vi "InitializeGenericCommandDialog.vi"(8 "Error In":errorcluster, 10 "Initial List Values":string[](array[string]), 11 "Dialog Enter Generic_UICtrlRefnums":T1) -> (0 "Error Out":errorcluster)   [LabVIEW 2012]
doc: "SciScan 1.2 160622"
uses:
  Dialog Enter Generic_UICtrlRefnums.ctl
  Custom Controls and Typedefs/BOOL Enum.ctl
  Custom Controls and Typedefs/Delete Button.ctl
  CommonResource VIs/UI Control and Indicator properties_Commands.ctl
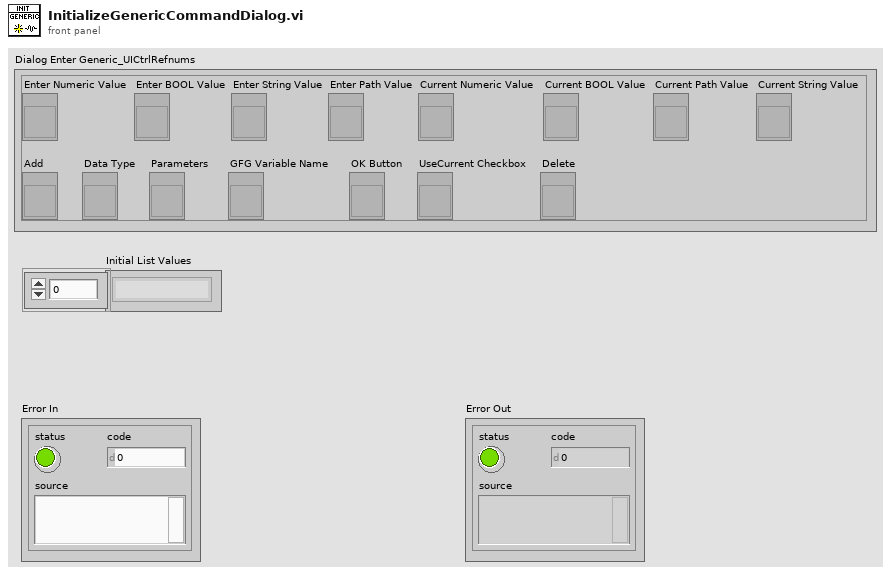
[diagram p1: front panel]
types:
  T1 = typedef "Dialog Enter Generic_UICtrlRefnums.ctl" = cluster{"Enter Numeric Value":refnum<vi>, "Enter BOOL Value":refnum<vi>, "Enter String Value":refnum<vi>, "Enter Path Value":refnum<vi>, "Add":refnum<vi>, "Data Type":refnum<vi>, "Parameters":refnum<vi>, "GFG Variable Name":refnum<vi>, "OK Button":refnum<vi>, "Current Numeric Value":refnum<vi>, "Current BOOL Value":refnum<vi>, "Current String Value":refnum<vi>, "Current Path Value":refnum<vi>, "UseCurrent Checkbox":refnum<vi>, "Delete":refnum<vi>}
  T2 = typedef "UI Control and Indicator properties_Commands.ctl" = enum16{"Enable", "Disable", "Disable and Grey", "Make Visible", "Make Invisible"}
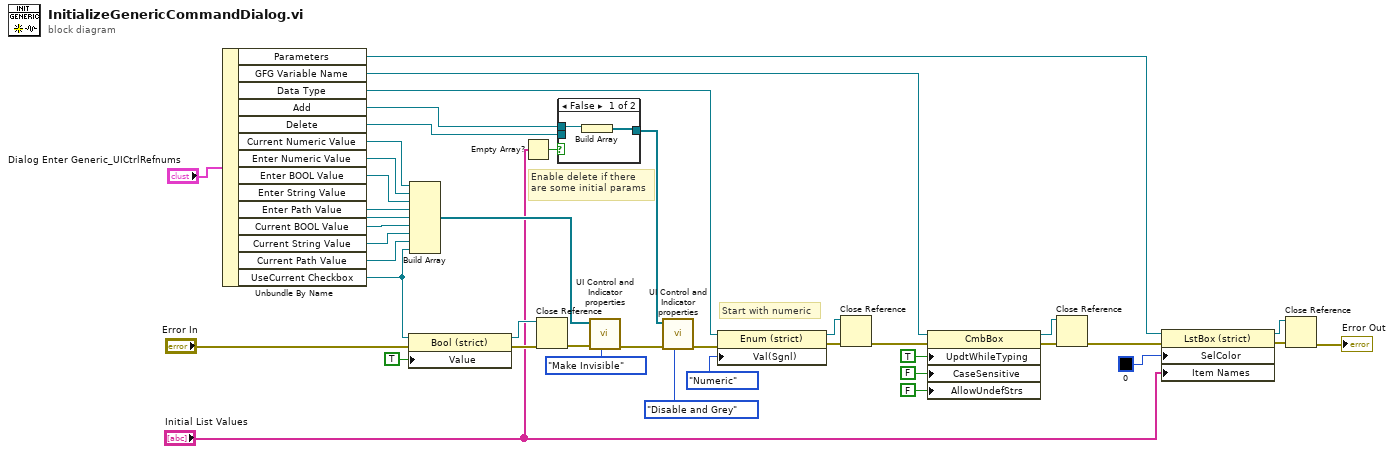
[diagram p0: block diagram]
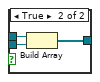
[diagram p2: hidden frame]
diagram:
  # "Enable delete if there\nare some initial params"
  # "Start with numeric"
  n1 = Unbundle By Name("Dialog Enter Generic_UICtrlRefnums") -> ("Parameters"=w16:refnum<vi>, "GFG Variable Name"=w29:refnum<vi>, "Data Type"=w37:refnum<vi>, "Add"=w26:refnum<vi>, "Delete"=w18:refnum<vi>, "Current Numeric Value"=w20:refnum<vi>, "Enter Numeric Value"=w21:refnum<vi>, "Enter BOOL Value"=w41:refnum<vi>, "Enter String Value"=w40:refnum<vi>, "Enter Path Value"=w39:refnum<vi>, "Current BOOL Value"=w24:refnum<vi>, "Current String Value"=w23:refnum<vi>, "Current Path Value"=w22:refnum<vi>, "UseCurrent Checkbox"=w8:refnum<vi>)
  n2 = property class="Bool (strict)"(reference=w8, error in="Error In", "Value"=TRUE) -> (reference out=w5:refnum<vi>, error out=w6:errorcluster)
  n3 = Build Array(w20, w21, w41, w40, w39, w24, w23, w22, w8) -> (w38:refnum<vi>[])
  n4 = Empty Array?(array="Initial List Values") -> (empty?=w1:bool)
  n5 = Close Reference(reference=w5, error in (no error)=w6) -> (error out=w4:errorcluster)
  n6 = case shown="False" w1 {
    tunnel: w26 -> [w44 w47]
    tunnel: [w43 w46] -> w25
    tunnel: w18 -> [_ w45]
    frame False {
      n7 = Build Array(w44) -> (w43:refnum<vi>[])
    }
    frame True {
      n8 = Build Array(w47, w45) -> (w46:refnum<vi>[])
    }
  }
  n9 = call "UI Control and Indicator properties.vi"("Enable Command"=UI_Control_and_Indicator_properties_Commands."Make Invisible", "Error In"=w4, "Control Refnums"=w38) -> ("Error Out"=w19:errorcluster)  [unwired: 8 in]
  n10 = call "UI Control and Indicator properties.vi"("Enable Command"=UI_Control_and_Indicator_properties_Commands."Disable and Grey", "Error In"=w19, "Control Refnums"=w25) -> ("Error Out"=w28:errorcluster)  [unwired: 8 in]
  n11 = property class="Enum (strict)"(reference=w37, error in=w28, "Val(Sgnl)"=enum16{"Numeric", "Boolean", "String", "Path"}."Numeric" ("Value")) -> (reference out=w34:refnum<vi>, error out=w35:errorcluster)
  n12 = Close Reference(reference=w34, error in (no error)=w35) -> (error out=w32:errorcluster)
  n13 = property class="CmbBox"(reference=w29, error in=w32, "UpdtWhileTyping"=TRUE ("Update While Typing?"), "CaseSensitive"=FALSE ("Case Sensitive Pop-up"), "AllowUndefStrs"=FALSE ("Allow Undefined Strings")) -> (reference out=w31:refnum<vi>, error out=w30:errorcluster)
  n14 = Close Reference(reference=w31, error in (no error)=w30) -> (error out=w15:errorcluster)
  n15 = property class="LstBox (strict)"(reference=w16, error in=w15, "SelColor"=u32 0, "Item Names"="Initial List Values") -> (reference out=w13:refnum<vi>, error out=w14:errorcluster)
  n16 = Close Reference(reference=w13, error in (no error)=w14) -> (error out=→"Error Out":errorcluster)
